vi "fetch_and_translate_trigger.vi"(8 "error in (no error)":errorcluster, 11 "ExperimentControllerDL090803Triggered in":refnum<class "ExperimentControllerDL090803Triggered.lvclass">) -> (0 "error out":errorcluster, 1 "sender TLC type":T1=enum."ImagingMode", 2 "statechart trigger":T2, 3 "ExperimentControllerDL090803Triggered out":refnum<class "ExperimentControllerDL090803Triggered.lvclass">)   [LabVIEW 2010, in "ExperimentControllerDL090803Triggered.lvclass"]
uses:
  ExperimentControllerDL090803Triggered.lvclass
  internal_trigger_enum.ctl
  common/enumerations/top-level_component_type_enum.ctl
  GenericExperimentController/GenericExperimentController/trigger_enum.ctl
  GenericExperimentController/GenericExperimentController/GenericExperimentController.lvclass
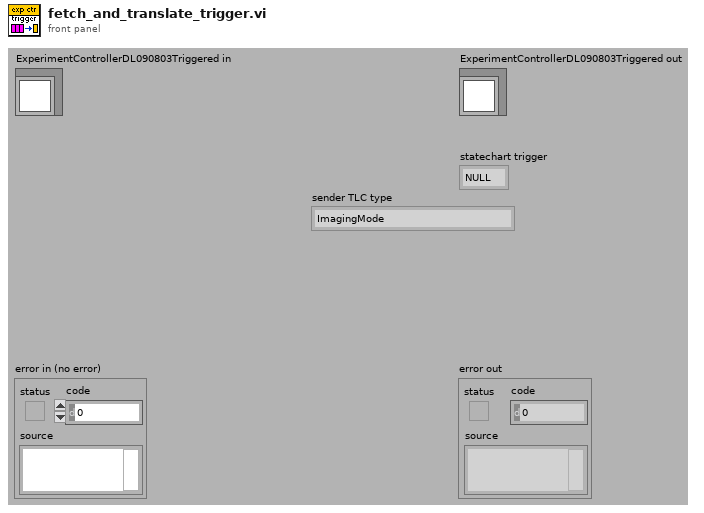
[diagram p1: front panel]
types:
  T1 = typedef "top-level_component_type_enum.ctl" = enum16{"undefined", "ImagingMode", "ScanHead", "DAQ", "ImageAssembler", "Display", "DataCollection", "Analyser", "Stimulator", "ExperimentController", "Instrument", "Stage"}
  T2 = typedef "ExperimentControllerDL090803Triggered.lvclass/internal_trigger_enum.ctl" = enum16{"NULL", "initialise", "terminate", "proceed", "start", "stop"}
  T3 = typedef "GenericExperimentController.lvclass/trigger_enum.ctl" = enum16{"NULL", "proceed", "prepare"}
  T4 = typedef "GenericToplevelComponent.lvclass/common_trigger_enum.ctl" = enum16{"NULL", "initialise", "terminate", "fetch command", "fetch data", "attach observer", "register as observer", "detach observer", "acknowledge", "start", "stop", "sweep started", "sweep finished", "experiment started", "experiment stopped"}
  T5 = typedef "trigger_type_enum.ctl" = enum8{"external", "internal", "common"}
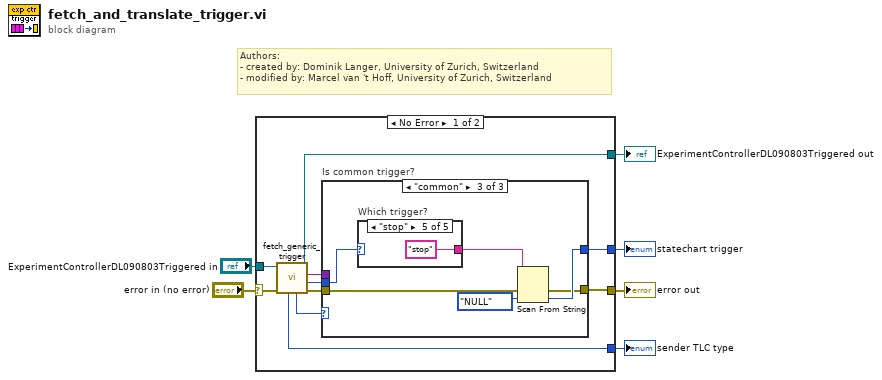
[diagram p0: block diagram]
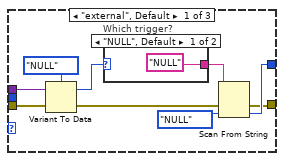
[diagram p2: hidden frame]
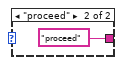
[diagram p3: hidden frame]
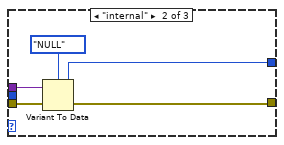
[diagram p4: hidden frame]
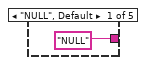
[diagram p5: hidden frame]
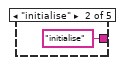
[diagram p6: hidden frame]
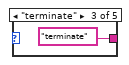
[diagram p7: hidden frame]
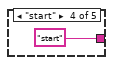
[diagram p8: hidden frame]
diagram:
  # "Authors: \n- created by: Dominik Langer, University of Zurich, Switzerland\n- modified by: Marcel van 't Hoff, University of Zurich, Switzerland"
  n1 = case shown="No Error" "error in (no error)" {
    selector: "error in (no error)" -> [w16 w45]
    tunnel: [w9 w45] -> w5
    tunnel: [w14 w44] -> w3
    tunnel: "ExperimentControllerDL090803Triggered in" -> [w15 w44]
    tunnel: [w8 _] -> w1
    tunnel: [w7 _] -> w2
    frame No Error {
      n2 = call-dynamic "fetch_generic_trigger.vi"("error in (no error)"=w16, "GenericToplevelComponent in"=w15) -> ("error out"=w10:errorcluster, "common trigger"=w12:T4, "trigger"=w11:variant, "GenericToplevelComponent out"=w14:refnum<class "ExperimentControllerDL090803Triggered.lvclass">, "trigger type"=w13:T5, "sender TLC type"=w7:T1)  [unwired: 3 in, 1 out]
      n3 = case "Is common trigger?" shown="\"common\"" w13 {
        tunnel: w12 -> [_ _ w38]
        tunnel: w11 -> [w22 w32 _]
        tunnel: w10 -> [w24 w31 w34]
        tunnel: [w17 w30 w33] -> w9
        tunnel: [w20 w29 w36] -> w8
        frame "external", Default {
          n4 = Variant To Data(error in=w24, Variant=w22, type=trigger_enum."NULL" ("trigger")) -> (error out=w18:errorcluster, data=w23:T3)
          n5 = case "Which trigger?" shown="\"NULL\", Default" w23 {
            tunnel: ["NULL" "proceed"] -> w19
            frame "NULL", Default {
            }
            frame "proceed" {
            }
          }
          n6 = Scan From String(input string=w19, error in=w18, default 1=internal_trigger_enum."NULL" ("statechart trigger")) -> (error out=w17:errorcluster, output 1=w20:T2)  [unwired: 2 in, 2 out]
        }
        frame "internal" {
          n7 = Variant To Data(error in=w31, Variant=w32, type=internal_trigger_enum."NULL" ("statechart trigger")) -> (error out=w30:errorcluster, data=w29:T2)
        }
        frame "common" {
          n8 = case "Which trigger?" shown="\"stop\"" w38 {
            tunnel: ["NULL" "initialise" "terminate" "start" "stop"] -> w35
            frame "NULL", Default {
            }
            frame "initialise" {
            }
            frame "terminate" {
            }
            frame "start" {
            }
            frame "stop" {
            }
          }
          n9 = Scan From String(input string=w35, error in=w34, default 1=internal_trigger_enum."NULL" ("statechart trigger")) -> (error out=w33:errorcluster, output 1=w36:T2)  [unwired: 2 in, 2 out]
        }
      }
    }
    frame Error {
    }
  }
  "error out" <- w5
  "ExperimentControllerDL090803Triggered out" <- w3
  "statechart trigger" <- w1
  "sender TLC type" <- w2
